vi "Write IO Card.vi"(5 "parity (0:none)":enum16{"None", "Odd", "Even", "Mark", "Space"}(ring), 6 "IO Card Function":T1, 7 "Check Info":string="OK", 8 "error in (no error)":errorcluster, 9 "write buffer":string, 10 "baud rate (9600)":u32=1000000, 11 "VISA resource name":refnum<visa-resource-name>) -> (0 "error out":errorcluster, 2 "read buffer":string, 3 "VISA resource name out":refnum<visa-resource-name>)   [LabVIEW 2020]
uses:
  subvi/IO Card Function Choose.ctl
  be62113c-601f-4bc0-9a60-b62963abe075.vi
  7a53a4da-c08b-4e64-bf64-35571d2fedff.vi
  <vilib>/Instr/_visa.llb/VISA Configure Serial Port (Instr).vi
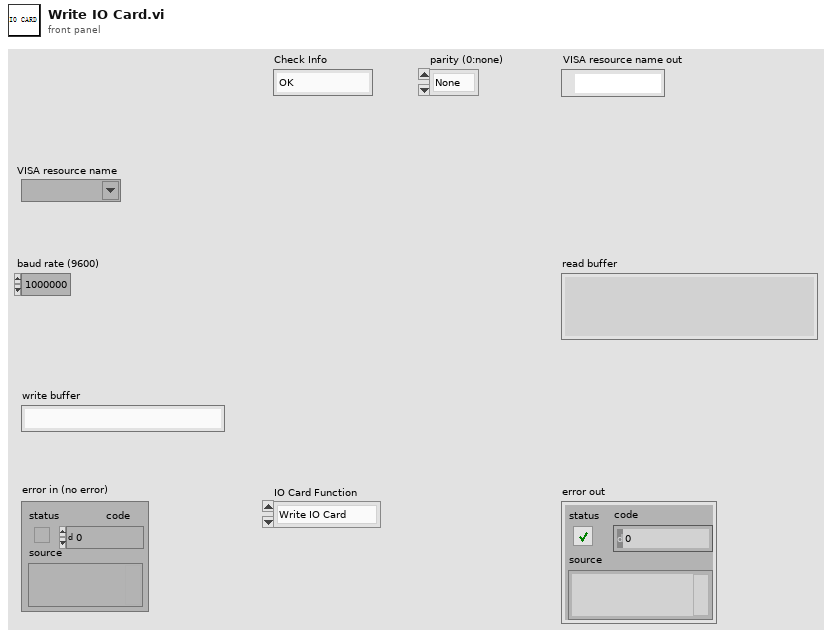
[diagram p1: front panel]
types:
  T1 = typedef "IO Card Function Choose.ctl" = enum16{"Write IO Card", "Init IO Card"}
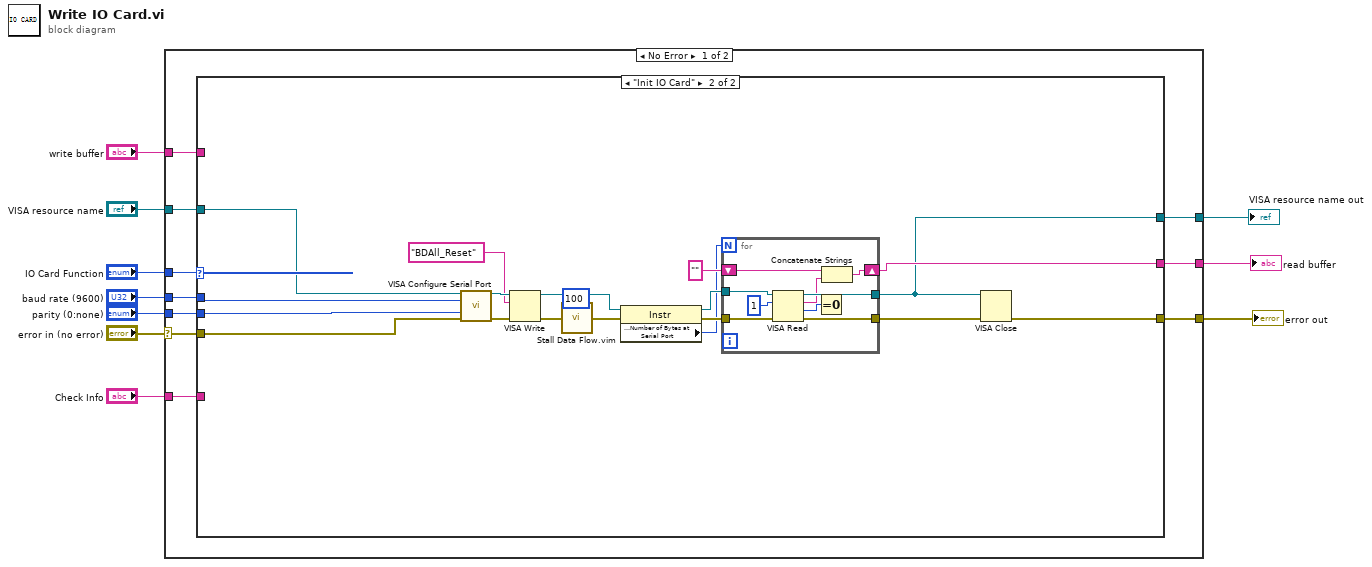
[diagram p0: block diagram]
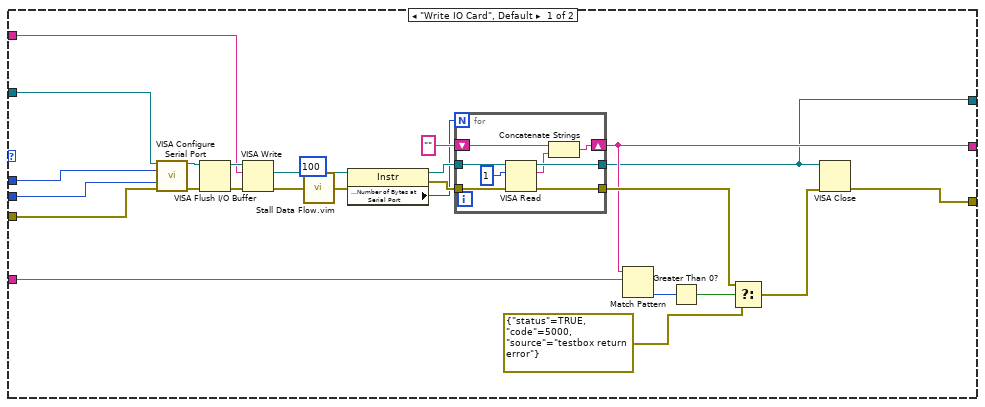
[diagram p2: hidden frame]
diagram:
  n1 = case shown="No Error" "error in (no error)" {
    selector: "error in (no error)" -> [w12 w83]
    tunnel: "IO Card Function" -> [w20 _]
    tunnel: [w19 w83] -> w9
    tunnel: [w18 _] -> w8
    tunnel: "VISA resource name" -> [w17 _]
    tunnel: "parity (0:none)" -> [w16 _]
    tunnel: "baud rate (9600)" -> [w15 _]
    tunnel: "write buffer" -> [w14 _]
    tunnel: "Check Info" -> [w13 _]
    tunnel: [w11 _] -> w1
    frame No Error {
      n2 = case shown="\"Init IO Card\"" w20 {
        tunnel: w12 -> [w22 w61]
        tunnel: [w25 w60] -> w19
        tunnel: [w26 w59] -> w18
        tunnel: w17 -> [w23 w58]
        tunnel: w16 -> [w29 w56]
        tunnel: w15 -> [w28 w57]
        tunnel: w14 -> [w27 _]
        tunnel: w13 -> [w24 _]
        tunnel: [w21 w55] -> w11
        frame "Write IO Card", Default {
          n3 = call-poly "VISA Configure Serial Port"("VISA resource name"=w23, "baud rate (9600)"=w28, "parity (0:none)"=w29, "error in (no error)"=w22) -> ("VISA resource name out"=w42:refnum<visa-resource-name>, "error out"=w43:errorcluster)  [unwired: 10 in]
          n4 = VISA Flush I/O Buffer(VISA resource name=w42, error in (no error)=w43) -> (VISA resource name out=w41:refnum<visa-resource-name>, error out=w40:errorcluster)  [unwired: 1 in]
          n5 = VISA Write(VISA resource name=w41, write buffer=w27, error in (no error)=w40) -> (VISA resource name out=w39:refnum<visa-resource-name>, error out=w46:errorcluster)  [unwired: 1 out]
          n6 = call "Stall Data Flow.vim"("value in"=w46, "milliseconds to wait"=u32 100) -> ("value out"=w37:errorcluster)  [unwired: 1 out]
          n7 = property class="Instr"(reference=w39, error in=w37) -> (reference out=w38:refnum<visa-resource-name>, error out=w36:errorcluster, "Serial Settings:Number of Bytes at Serial Port"=w35:u32)
          n8 = for {
            N: w35 -> [_]
            shift-right: [w51] -> w26
            shift-left: "" -> [w52]
            tunnel: w38 -> [w50]
            tunnel: [w54] -> w21
            tunnel: w36 -> [w49]
            tunnel: [w53] -> w30
            n9 = VISA Read(VISA resource name=w50, byte count=u32 1, error in (no error)=w49) -> (VISA resource name out=w54:refnum<visa-resource-name>, read buffer=w47:string, error out=w53:errorcluster)  [unwired: 1 out]
            n10 = Concatenate Strings(w52, w47) -> (w51:string)
          }
          n11 = Match Pattern(string=w26, regular expression=w24) -> (offset past match=w34:i32)  [unwired: 1 in, 3 out]
          n12 = Greater Than 0?(x=w34) -> (x > 0?=w33:bool)
          n13 = Select(t=w30, s=w33, f=errorcluster {"status"=TRUE, "code"=5000, "source"="testbox return error"}) -> (s? t:f=w31:errorcluster)
          n14 = VISA Close(VISA resource name=w21, error in (no error)=w31) -> (error out=w25:errorcluster)
        }
        frame "Init IO Card" {
          n15 = call-poly "VISA Configure Serial Port"("VISA resource name"=w58, "baud rate (9600)"=w57, "parity (0:none)"=w56, "error in (no error)"=w61) -> ("VISA resource name out"=w73:refnum<visa-resource-name>, "error out"=w72:errorcluster)  [unwired: 10 in]
          n16 = VISA Write(VISA resource name=w73, write buffer="BDAll_Reset", error in (no error)=w72) -> (VISA resource name out=w66:refnum<visa-resource-name>, error out=w70:errorcluster)  [unwired: 1 out]
          n17 = call "Stall Data Flow.vim"("value in"=w70, "milliseconds to wait"=u32 100) -> ("value out"=w64:errorcluster)  [unwired: 1 out]
          n18 = property class="Instr"(reference=w66, error in=w64) -> (reference out=w65:refnum<visa-resource-name>, error out=w63:errorcluster, "Serial Settings:Number of Bytes at Serial Port"=w62:u32)
          n19 = for {
            N: w62 -> [_]
            shift-right: [w79] -> w59
            shift-left: "" -> [w78]
            tunnel: [w82] -> w55
            tunnel: w63 -> [w80]
            tunnel: [w81] -> w71
            tunnel: w65 -> [w74]
            n20 = VISA Read(VISA resource name=w74, byte count=u32 1, error in (no error)=w80) -> (VISA resource name out=w82:refnum<visa-resource-name>, read buffer=w75:string, return count=w76:u32, error out=w81:errorcluster)
            n21 = Equal To 0?(x=w76) -> ()  [unwired: 1 out]
            n22 = Concatenate Strings(w78, w75) -> (w79:string)
          }
          n23 = VISA Close(VISA resource name=w55, error in (no error)=w71) -> (error out=w60:errorcluster)
        }
      }
    }
    frame Error {
    }
  }
  "error out" <- w9
  "read buffer" <- w8
  "VISA resource name out" <- w1
